vi "Set Control Font.vi"(4 "Error In":errorcluster, 6 "Font Parameters":T1, 7 "Font Settting in":refnum<class "Display Properties_WaveformChart.lvclass">) -> (0 "Error Out":errorcluster, 3 "Font Settting out":refnum<class "Display Properties_WaveformChart.lvclass">)   [LabVIEW 2015, in "Display Properties Manager.lvlib" / "Display Properties_WaveformChart.lvclass"]
uses:
  Display Properties_WaveformChart.lvclass
  _typedefs/Font Parameters.ctl
  _typedefs/Control Component to Set.ctl
  Display Properties.lvclass
  Display Properties Manager.lvlib
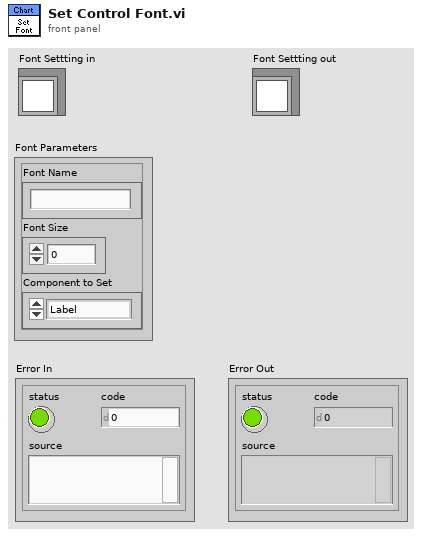
[diagram p1: front panel]
types:
  T1 = typedef "Display Properties Manager.lvlib/Font Parameters.ctl" = cluster{"Font Name":string, "Font Size":u32, "Component to Set":T2}
  T2 = typedef "Display Properties Manager.lvlib/Control Component to Set.ctl" = enum16{"Label", "Caption", "Contents"}
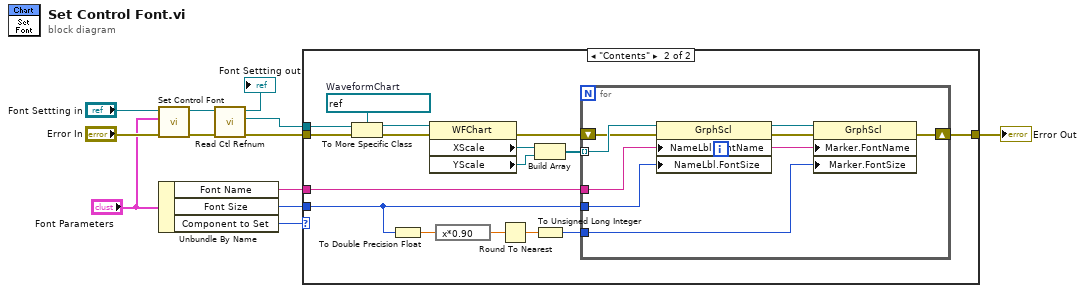
[diagram p0: block diagram]
diagram:
  n1 = call-parent "Set Control Font.vi"("Error In"="Error In", "Font Parameters"="Font Parameters", "Font Settting in"="Font Settting in") -> ("Error Out"=w9:errorcluster, "Font Settting out"=w10:refnum<class "Display Properties_WaveformChart.lvclass">)  [unwired: 3 in]
  n2 = Unbundle By Name("Font Parameters") -> ("Font Name"=w2:string, "Font Size"=w1:u32, "Component to Set"=w4:T2)
  n3 = call-dynamic "Read Ctl Refnum.vi"("Error In"=w9, "Font Settting in"=w10) -> ("Error Out"=w7:errorcluster, "Ctl Refnum"=w3:refnum<vi>, "Font Settting out"=→"Font Settting out":refnum<class "Display Properties_WaveformChart.lvclass">)  [unwired: 3 in]
  n4 = case shown="\"Contents\"" w4 {
    tunnel: w7 -> [w13 w29]
    tunnel: [w13 w19] -> w6
    tunnel: w3 -> [_ w27]
    tunnel: w2 -> [_ w20]
    tunnel: w1 -> [_ w15]
    frame Default {
    }
    frame "Contents" {
      w25 = refnum<vi> refnum  # WaveformChart
      n5 = To More Specific Class(target class=w25, reference=w27, error in=w29) -> (specific class reference=w26:refnum<vi>, error out=w28:errorcluster)
      n6 = To Double Precision Float(number=w15) -> (double precision float=w16:dbl)
      n7 = property class="WFChart"(reference=w26, error in=w28) -> (error out=w21:errorcluster, "XScale"=w24:refnum<vi>, "YScale"=w23:refnum<vi>)  [unwired: 1 out]
      n8 = expression code="x*0.90"(w16) -> (w17:dbl)
      n9 = Round To Nearest(number=w17) -> (nearest integer value=w18:dbl)
      n10 = Build Array(w24, w23) -> (w22:refnum<vi>[])
      n11 = To Unsigned Long Integer(number=w18) -> (unsigned 32bit integer=w14:u32)
      n12 = for {
        tunnel: w22 -> [w37] mode=indexing
        tunnel: w20 -> [w33]
        tunnel: w15 -> [w31]
        shift-right: [w32] -> w19
        shift-left: w21 -> [w36]
        tunnel: w14 -> [w30]
        n13 = property class="GrphScl"(reference=w37, error in=w36, "NameLbl.FontName"=w33, "NameLbl.FontSize"=w31) -> (reference out=w34:refnum<vi>, error out=w35:errorcluster)
        n14 = property class="GrphScl"(reference=w34, error in=w35, "Marker.FontName"=w33, "Marker.FontSize"=w30) -> (error out=w32:errorcluster)  [unwired: 1 out]
      }
    }
  }
  "Error Out" <- w6
